vi "CMDSendToBOX.vi"(8 "arg2":u16, 9 "arg1":u16, 10 "CMD":i8, 11 "VISA resource name":refnum<visa-resource-name>) -> (3 "VISA resource name out":refnum<visa-resource-name>)   [LabVIEW 2017]
panel:
  out "output array":u8[](array[numeric])
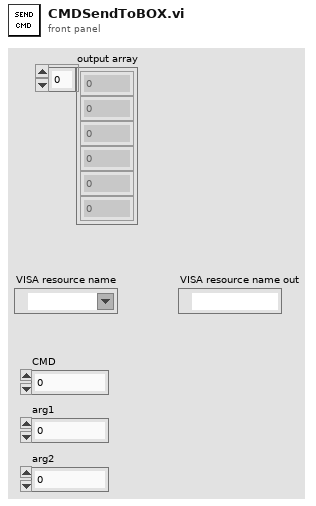
[diagram p1: front panel]
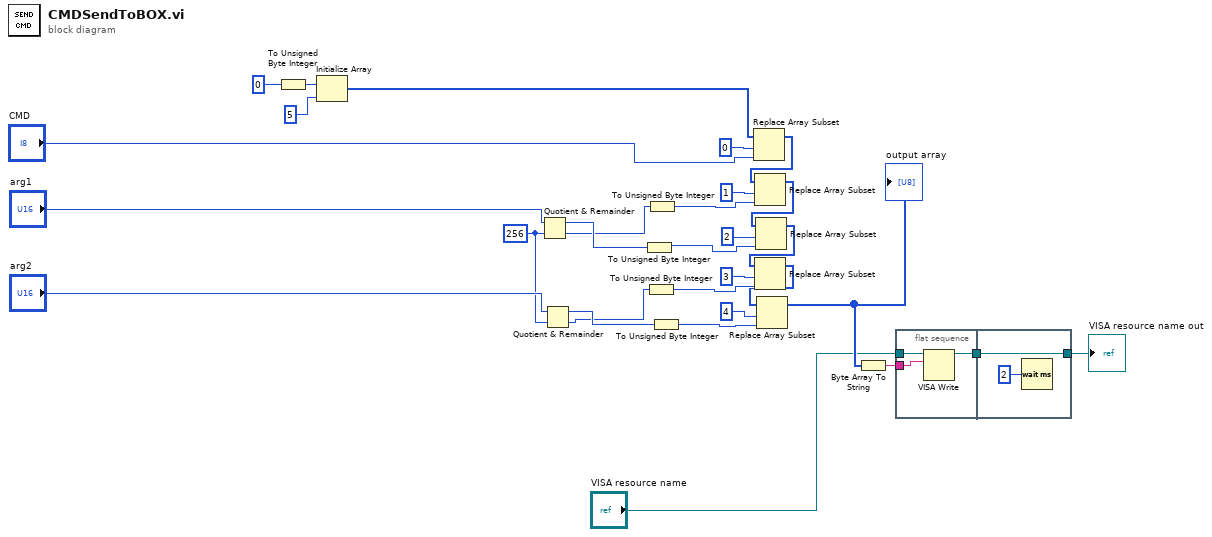
[diagram p0: block diagram]
diagram:
  w1 = u16 256 ("y")
  n1 = To Unsigned Byte Integer(number=u8 0) -> (unsigned 8bit integer=w9:u8)
  n2 = Initialize Array(w9, 5 ("dimension size")) -> (w7:u8[])
  n3 = Quotient & Remainder(x="arg1", y=w1) -> (x-y*floor(x/y)=w18:u16, floor(x/y)=w17:u16)
  n4 = Quotient & Remainder(x="arg2", y=w1) -> (x-y*floor(x/y)=w16:u16, floor(x/y)=w15:u16)
  n5 = To Unsigned Byte Integer(number=w18) -> (unsigned 8bit integer=w23:u8)
  n6 = To Unsigned Byte Integer(number=w15) -> (unsigned 8bit integer=w22:u8)
  n7 = To Unsigned Byte Integer(number=w17) -> (unsigned 8bit integer=w24:u8)
  n8 = To Unsigned Byte Integer(number=w16) -> (unsigned 8bit integer=w21:u8)
  n9 = Replace Array Subset(array=w7, new element="CMD", index=0) -> (w14:u8[])
  n10 = Replace Array Subset(array=w14, new element=w24, index=1) -> (w13:u8[])
  n11 = Replace Array Subset(array=w13, new element=w23, index=2) -> (w12:u8[])
  n12 = Replace Array Subset(array=w12, new element=w22, index=3) -> (w11:u8[])
  n13 = Replace Array Subset(array=w11, new element=w21, index=4) -> (w10:u8[])
  "output array" <- w10
  n14 = Byte Array To String(unsigned byte array=w10) -> (string=w3:string)
  n15 = flat-sequence {
    tunnel: "VISA resource name" -> [w33]
    tunnel: [w32] -> w4
    tunnel: w3 -> [w31]
    tunnel: [w34] -> w6
    tunnel: w4 -> [w34]
    frame #0 {
      n16 = VISA Write(VISA resource name=w33, write buffer=w31) -> (VISA resource name out=w32:refnum<visa-resource-name>)  [unwired: 1 in, 2 out]
    }
    frame #1 {
      n17 = Wait (ms)(milliseconds to wait=u32 2) -> ()  [unwired: 1 out]
    }
  }
  "VISA resource name out" <- w6
